vi "WzNetRem_Example_RAWprocess.vi"() -> ()   [LabVIEW 2012]
uses:
  Wizzler_NetworkRemoteToolkit.lvlib
panel:
  out "Signal Goodness":cluster{"Value":dbl, "Warning":string} {"Value" scale=0.9..2.0}
  out "Signal Level":cluster{"Value":dbl, "Warning":string} {"Value" scale=0.0..65535.0}
  out "Spectral Data":cluster{ext[], "Phase":dbl[]}[](graph)
  out "RAW interferogram":cluster{"Time":dbl[], "Intensity":dbl[]}(graph)
  out "Time profile":cluster{"Time":dbl[], "Intensity":dbl[]}[](graph)
  out "Numerics":T1={"Autoco duration FWHM"=0.0, "FTL time width FWHM"=nan, "TBP FWHM"=nan, "Spectral width FWHM"=nan, "Time width FWHM"=nan, "Mean wavelength"=nan, "Time stand. dev."=nan, "FTL time stand. dev."=nan, "Mean freq"=nan, "Spectral stand. dev."=nan, "TBP stand. dev."=nan, "Spectral width FWHM - nu"=nan, "Spectral stand. dev. - nu"=nan} {"Spectral stand. dev. - nu" format="%#.1f"; "Spectral width FWHM - nu" format="%#.1f"; "TBP stand. dev." format="%#.3f"; "Spectral stand. dev." format="%#.1f"; "Mean freq" format="%#.1f"; "FTL time stand. dev." format="%#.1f"; "Time stand. dev." format="%#.1f"; "Mean wavelength" format="%#.1f"; "Time width FWHM" format="%#.1f"; "Spectral width FWHM" format="%#.1f"; "TBP FWHM" format="%#.3f"; "FTL time width FWHM" format="%#.1f"}
  out "Acquisition TimeStamp":timestamp
  out "Read Spectral Data":dbl[][](array[numeric])
  in  "Path":path
  out "error out":errorcluster
  in  "machine name":string="127.0.0.1" caption="machine name (\"\":  open local reference)"
  in  "port number":u16=54321
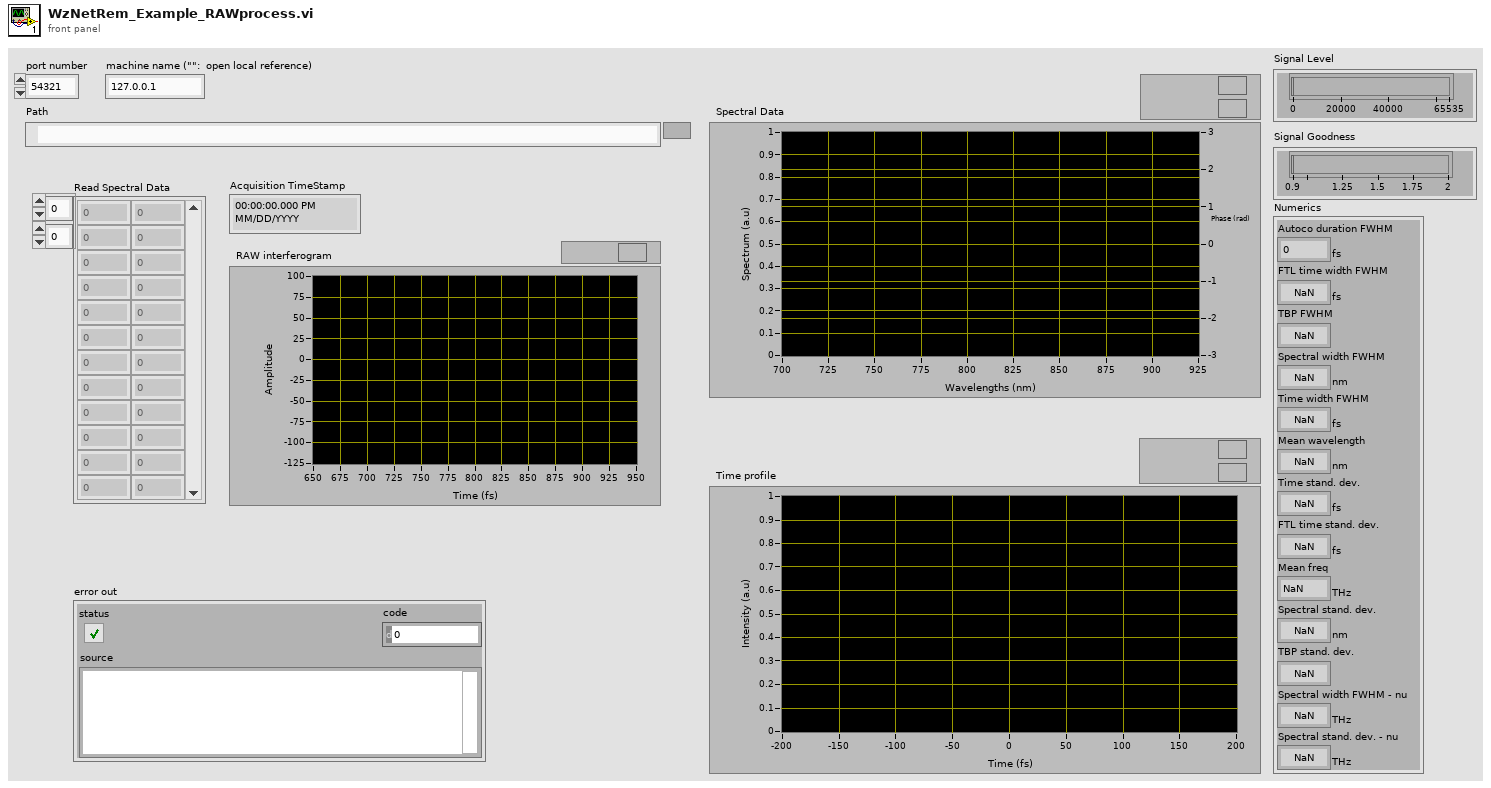
[diagram p1: front panel]
types:
  T1 = cluster{"Autoco duration FWHM":dbl[unit], "FTL time width FWHM":dbl[unit], "TBP FWHM":dbl, "Spectral width FWHM":dbl[unit], "Time width FWHM":dbl[unit], "Mean wavelength":dbl[unit], "Time stand. dev.":dbl[unit], "FTL time stand. dev.":dbl[unit], "Mean freq":dbl[unit], "Spectral stand. dev.":dbl[unit], "TBP stand. dev.":dbl, "Spectral width FWHM - nu":dbl[unit], "Spectral stand. dev. - nu":dbl[unit]}
  T2 = cluster{"Spectral profile":cluster{"Freq":dbl[], "Spectrum":dbl[], "Phase":dbl[], "Fit":dbl[], "Clipping mask":cluster{"start_index":i32, "width":i32}}, "Phase fit":cluster{"Ctrl freq":dbl[unit], "Poly. fit Coeffs.":dbl[]}, "Time profile":cluster{"Time":dbl[], "Intensity":dbl[], "Phase":dbl[]}, "Numerics":cluster{"Autoco duration FWHM":dbl[unit], "FTL time width FWHM":dbl[unit], "TBP FWHM":dbl, "Spectral width FWHM":dbl[unit], "Time width FWHM":dbl[unit], "Mean wavelength":dbl[unit], "Time stand. dev.":dbl[unit], "FTL time stand. dev.":dbl[unit], "Mean freq":dbl[unit], "Spectral stand. dev.":dbl[unit], "TBP stand. dev.":dbl, "Spectral width FWHM - nu":dbl[unit], "Spectral stand. dev. - nu":dbl[unit]}, "Time stamp":string, "Signal Quality":cluster{"Level":cluster{"Value":dbl, "String":string}, "Goodness":cluster{"Value":dbl, "String":string}, "Disable Num Displays":bool}}
  T3 = cluster{"Measured":cluster{"Time":dbl[], "Intensity":dbl[]}, "FTL":cluster{"Time":dbl[], "Intensity":dbl[]}}
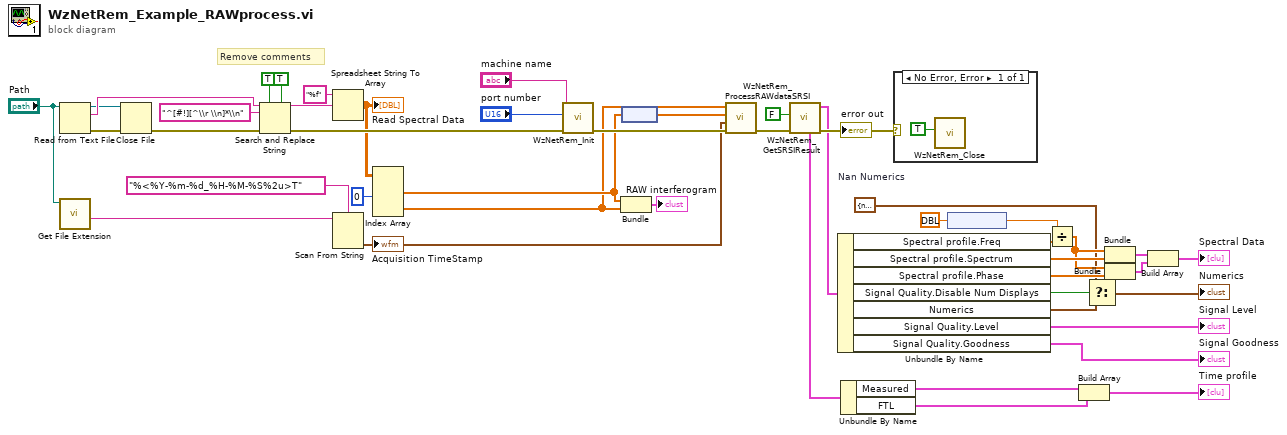
[diagram p0: block diagram]
diagram:
  w1 = T1 {"Autoco duration FWHM"=nan, "FTL time width FWHM"=nan, "TBP FWHM"=nan, "Spectral width FWHM"=nan, "Time width FWHM"=nan, "Mean wavelength"=nan, "Time stand. dev."=nan, "FTL time stand. dev."=nan, "Mean freq"=nan, "Spectral stand. dev."=nan, "TBP stand. dev."=nan, "Spectral width FWHM - nu"=nan, "Spectral stand. dev. - nu"=nan}  # Nan Numerics
  # "Remove comments"
  n1 = Read from Text File(file (use dialog)="Path") -> (refnum out=w41:refnum<file>, text=w44:string, error out=w42:errorcluster)  [unwired: 3 in, 1 out]
  n2 = call <vilib>:"Get File Extension.vi"("file"="Path") -> ("filename without extension"=w36:string)  [unwired: 7 in, 3 out]
  n3 = Close File(refnum=w41, error in=w42) -> (error out=w40:errorcluster)  [unwired: 1 out]
  n4 = Search and Replace String(replace all?=TRUE ("replace all? (F)"), multiline?=TRUE ("multiline? (F)"), input string=w44, search string="^[#!][^\\r \\n]*\\n", error in=w40) -> (result string=w39:string, error out=w31:errorcluster)  [unwired: 3 in, 2 out]
  n5 = Spreadsheet String To Array(format string="%f", spreadsheet string=w39) -> (array=w28:dbl[][])  [unwired: 2 in]
  "Read Spectral Data" <- w28
  n6 = Scan From String(format string="%<%Y-%m-%d_%H-%M-%S%2u>T", input string=w36) -> (output 1=w29:timestamp)  [unwired: 3 in, 3 out]
  "Acquisition TimeStamp" <- w29
  n7 = Index Array(array=w28, index (col) #1=0 ("disabled index (col)")) -> (element #1=w22:dbl[], element #2=w21:dbl[])  [unwired: 3 in]
  n8 = call "WzNetRem_Init.vi"("error in (no error)"=w31, "port number"="port number", "machine name"="machine name") -> ("error out"=w30:errorcluster)  [unwired: 8 in]
  n9 = Bundle(w22, w21) -> (→"RAW interferogram":cluster{dbl[], dbl[]})  [unwired: 1 in]
  n10 = node(w22) -> (w26:dbl[unit][])
  n11 = call "WzNetRem_ProcessRAWdataSRSI.vi"("error in (no error)"=w30, "TimeStamp"=w29, "Lambdas"=w26, "Raw spectrum"=w21) -> ("error out"=w25:errorcluster)  [unwired: 7 in]
  n12 = call "WzNetRem_GetSRSIResult.vi"("error in (no error)"=w25, "Ignore Old Results?"=FALSE ("Wait for next measurement?")) -> ("error out"=w24:errorcluster, "Num Results"=w4:T2, "Time Intensities"=w23:T3)  [unwired: 4 in, 3 out]
  "error out" <- w24
  n13 = Unbundle By Name(w4) -> ("Spectral profile.Freq"=w15:dbl[], "Spectral profile.Spectrum"=w16:dbl[], "Spectral profile.Phase"=w14:dbl[], "Signal Quality.Disable Num Displays"=w7:bool, "Numerics"=w11:T1, "Signal Quality.Level"=→"Signal Level":cluster{"Value":dbl, "String":string}, "Signal Quality.Goodness"=→"Signal Goodness":cluster{"Value":dbl, "String":string})
  n14 = Unbundle By Name(w23) -> ("Measured"=w19:cluster{"Time":dbl[], "Intensity":dbl[]}, "FTL"=w18:cluster{"Time":dbl[], "Intensity":dbl[]})
  n15 = case shown="No Error, Error" w24 {
    frame No Error {
      n16 = call "WzNetRem_Close.vi"("Force Meas. Stop"=TRUE) -> ()  [unwired: 10 in, 1 out]
    }
  }
  n17 = node(ext[unit] 299792458.0) -> (w8:ext)
  n18 = Divide(x=w8, y=w15) -> (x/y=w9:ext[])
  n19 = Build Array(w19, w18) -> (→"Time profile":cluster{"Time":dbl[], "Intensity":dbl[]}[])
  n20 = Select(t=w1, s=w7, f=w11) -> (s? t:f=→"Numerics":T1)
  n21 = Bundle(w9, "Spectrum"=w16) -> (w13:cluster{ext[], "Spectrum":dbl[]})  [unwired: 1 in]
  n22 = Bundle(w9, "Phase"=w14) -> (w12:cluster{ext[], "Phase":dbl[]})  [unwired: 1 in]
  n23 = Build Array(w13, w12) -> (→"Spectral Data":cluster{ext[], "Phase":dbl[]}[])
